vi "OdorSystem-V2.1.vi"() -> ()   [LabVIEW 2019]
doc: "Control odor delivery system in Setup B\n\nNeeds Labview 2019 and DAQmx 19! So that it is compatible with scanimage on Setup B\n\nBy Dr. Jan Eckhardt, Group Friedrich, FMI Basel"
uses:
  StatesEnum.ctl
  <vilib>/Utility/error.llb/DialogType.ctl
  <vilib>/DAQmx/write.llb/DAQmx Write (Digital 1D Bool NChan 1Samp 1Line).vi
  <vilib>/DAQmx/write.llb/DAQmx Write (Digital Wfm 1Chan NSamp).vi
  <vilib>/DAQmx/read.llb/DAQmx Read (Counter U32 1Chan 1Samp).vi
  <vilib>/DAQmx/read.llb/DAQmx Read (Digital 1D Bool 1Chan 1Samp).vi
  <vilib>/Utility/config.llb/Read Key (Double).vi
  <vilib>/Utility/config.llb/Read Key (I32).vi
  <vilib>/Utility/config.llb/Read Key (Boolean).vi
  <vilib>/Utility/config.llb/Read Key (String).vi
  <vilib>/DAQmx/miscellaneous.llb/DAQmx Fill In Error Info.vi
  <vilib>/DAQmx/create/channels.llb/DAQmx Create Channel (CO-Pulse Generation-Frequency).vi
  <vilib>/Waveform/DWDTOps.llb/Digital Pattern Generator (Single Value).vi
  <vilib>/Waveform/DWDTOps.llb/DWDT Append Digital Samples.vi
  <vilib>/DAQmx/configure/timing.llb/DAQmx Timing (Implicit).vi
  <vilib>/DAQmx/create/channels.llb/DAQmx Create Channel (CI-Count Edges).vi
  <vilib>/DAQmx/configure/timing.llb/DAQmx Timing (Sample Clock).vi
  <vilib>/Waveform/DWDTOps.llb/DWDT Append Digital Signals.vi
  <vilib>/Waveform/DWDTOps.llb/DWDT Digital to Boolean Array.vi
  <vilib>/DAQmx/create/channels.llb/DAQmx Create Channel (DO-Digital Output).vi
  <vilib>/Waveform/DWDTOps.llb/DWDT Uncompress Digital.vi
  <resource>/objmgr/daqmx.rc
  <vilib>/Utility/config.llb/NI_LVConfig.lvlib
panel:
  out "Loaded experiment":string
  in  "Load exp. ini":bool
  in  "Use Default valve":bool=TRUE
  in  "Selected default valve":u8(knob)=8 min=1 max=8 step=1 scale=1.0..8.0
  out "Framecount":u32
  in  "Image count filepath":path
  out "Experiment running":bool
  out "State":T1
  in  "Select experiment":enum32{"Single trial", "Trial series"}(tab)
  out "Time elapsed":dbl format="%.1f"
  in  "Start single trial":bool
  out "single trial done":bool
  in  "Select valve":u8(knob)=1 min=1 max=8 step=1 scale=1.0..8.0
  out "Pause elapsed time":dbl format="%#.1f"
  out "In between trials":bool
  out "Trial elapsed time":dbl format="%.1f"
  out "Total elapsed time":dbl format="%.1f"
  out "Estimated total time":dbl
  out "Current list index":i32
  out "Current Valve":u8
  in  "Time between trials":u16=10 min=1 max=900 step=1
  in  "Start trial series":bool
  in  "Valve order list":i8[](array[numeric]) min=1 max=8 step=1
  out "Digitaler output":digitalwaveform(graph)
  out "Stop Boolesch":bool
  in  "Total trial time":dbl=20.0 min=1.0 step=0.1
  in  "Valve opening time":dbl=10.0 min=0.0 step=0.1
  in  "Valve delay":dbl=2.0 min=0.0 step=0.1
  in  "Stopp":bool
  out "Digital Waveform Graph":digitalwaveform(graph)
  # "All times are in second!"
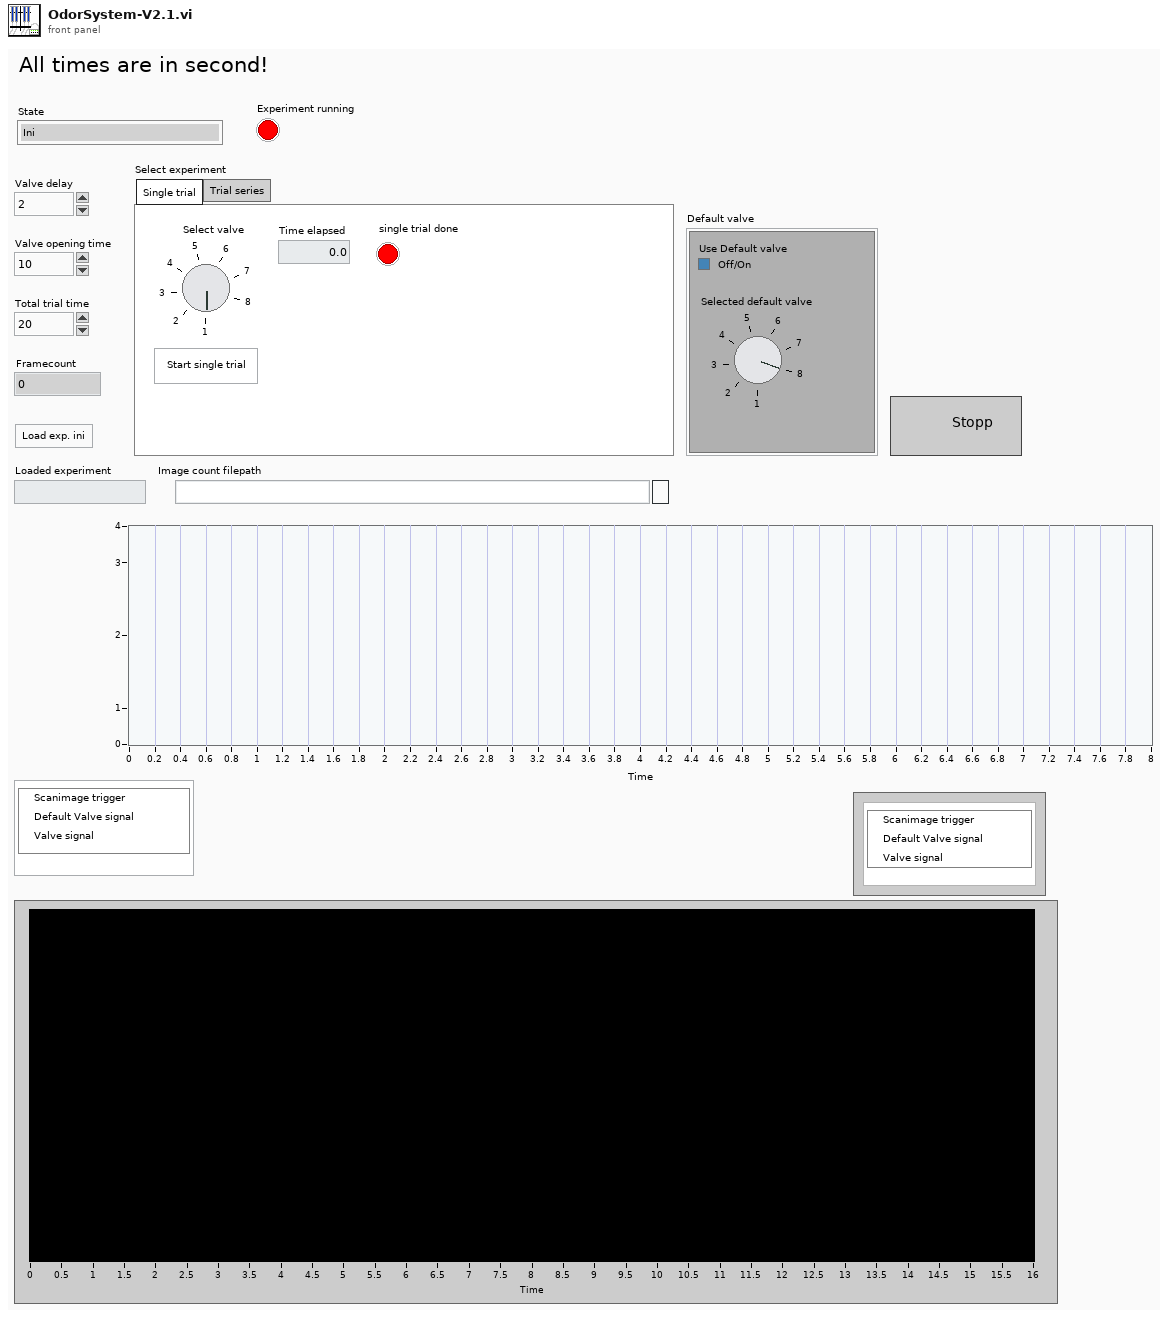
[diagram p1: front panel]
types:
  T1 = typedef "StatesEnum.ctl" = enum16{"Ini", "Standby", "Start Trial", "Start trial series", "Stop"}
  T2 = enum8{"Enabled", "Disabled", "Disabled and Grayed Out"}
  T3 = enum32{"Page Enabled", "Page Disabled", "Page Disabled & Grayed"}
  T4 = typedef "NI_LVConfig.lvlib/Config Data RefNum.ctl" = refnum<k1>
  T5 = typedef "DialogType.ctl" = u16
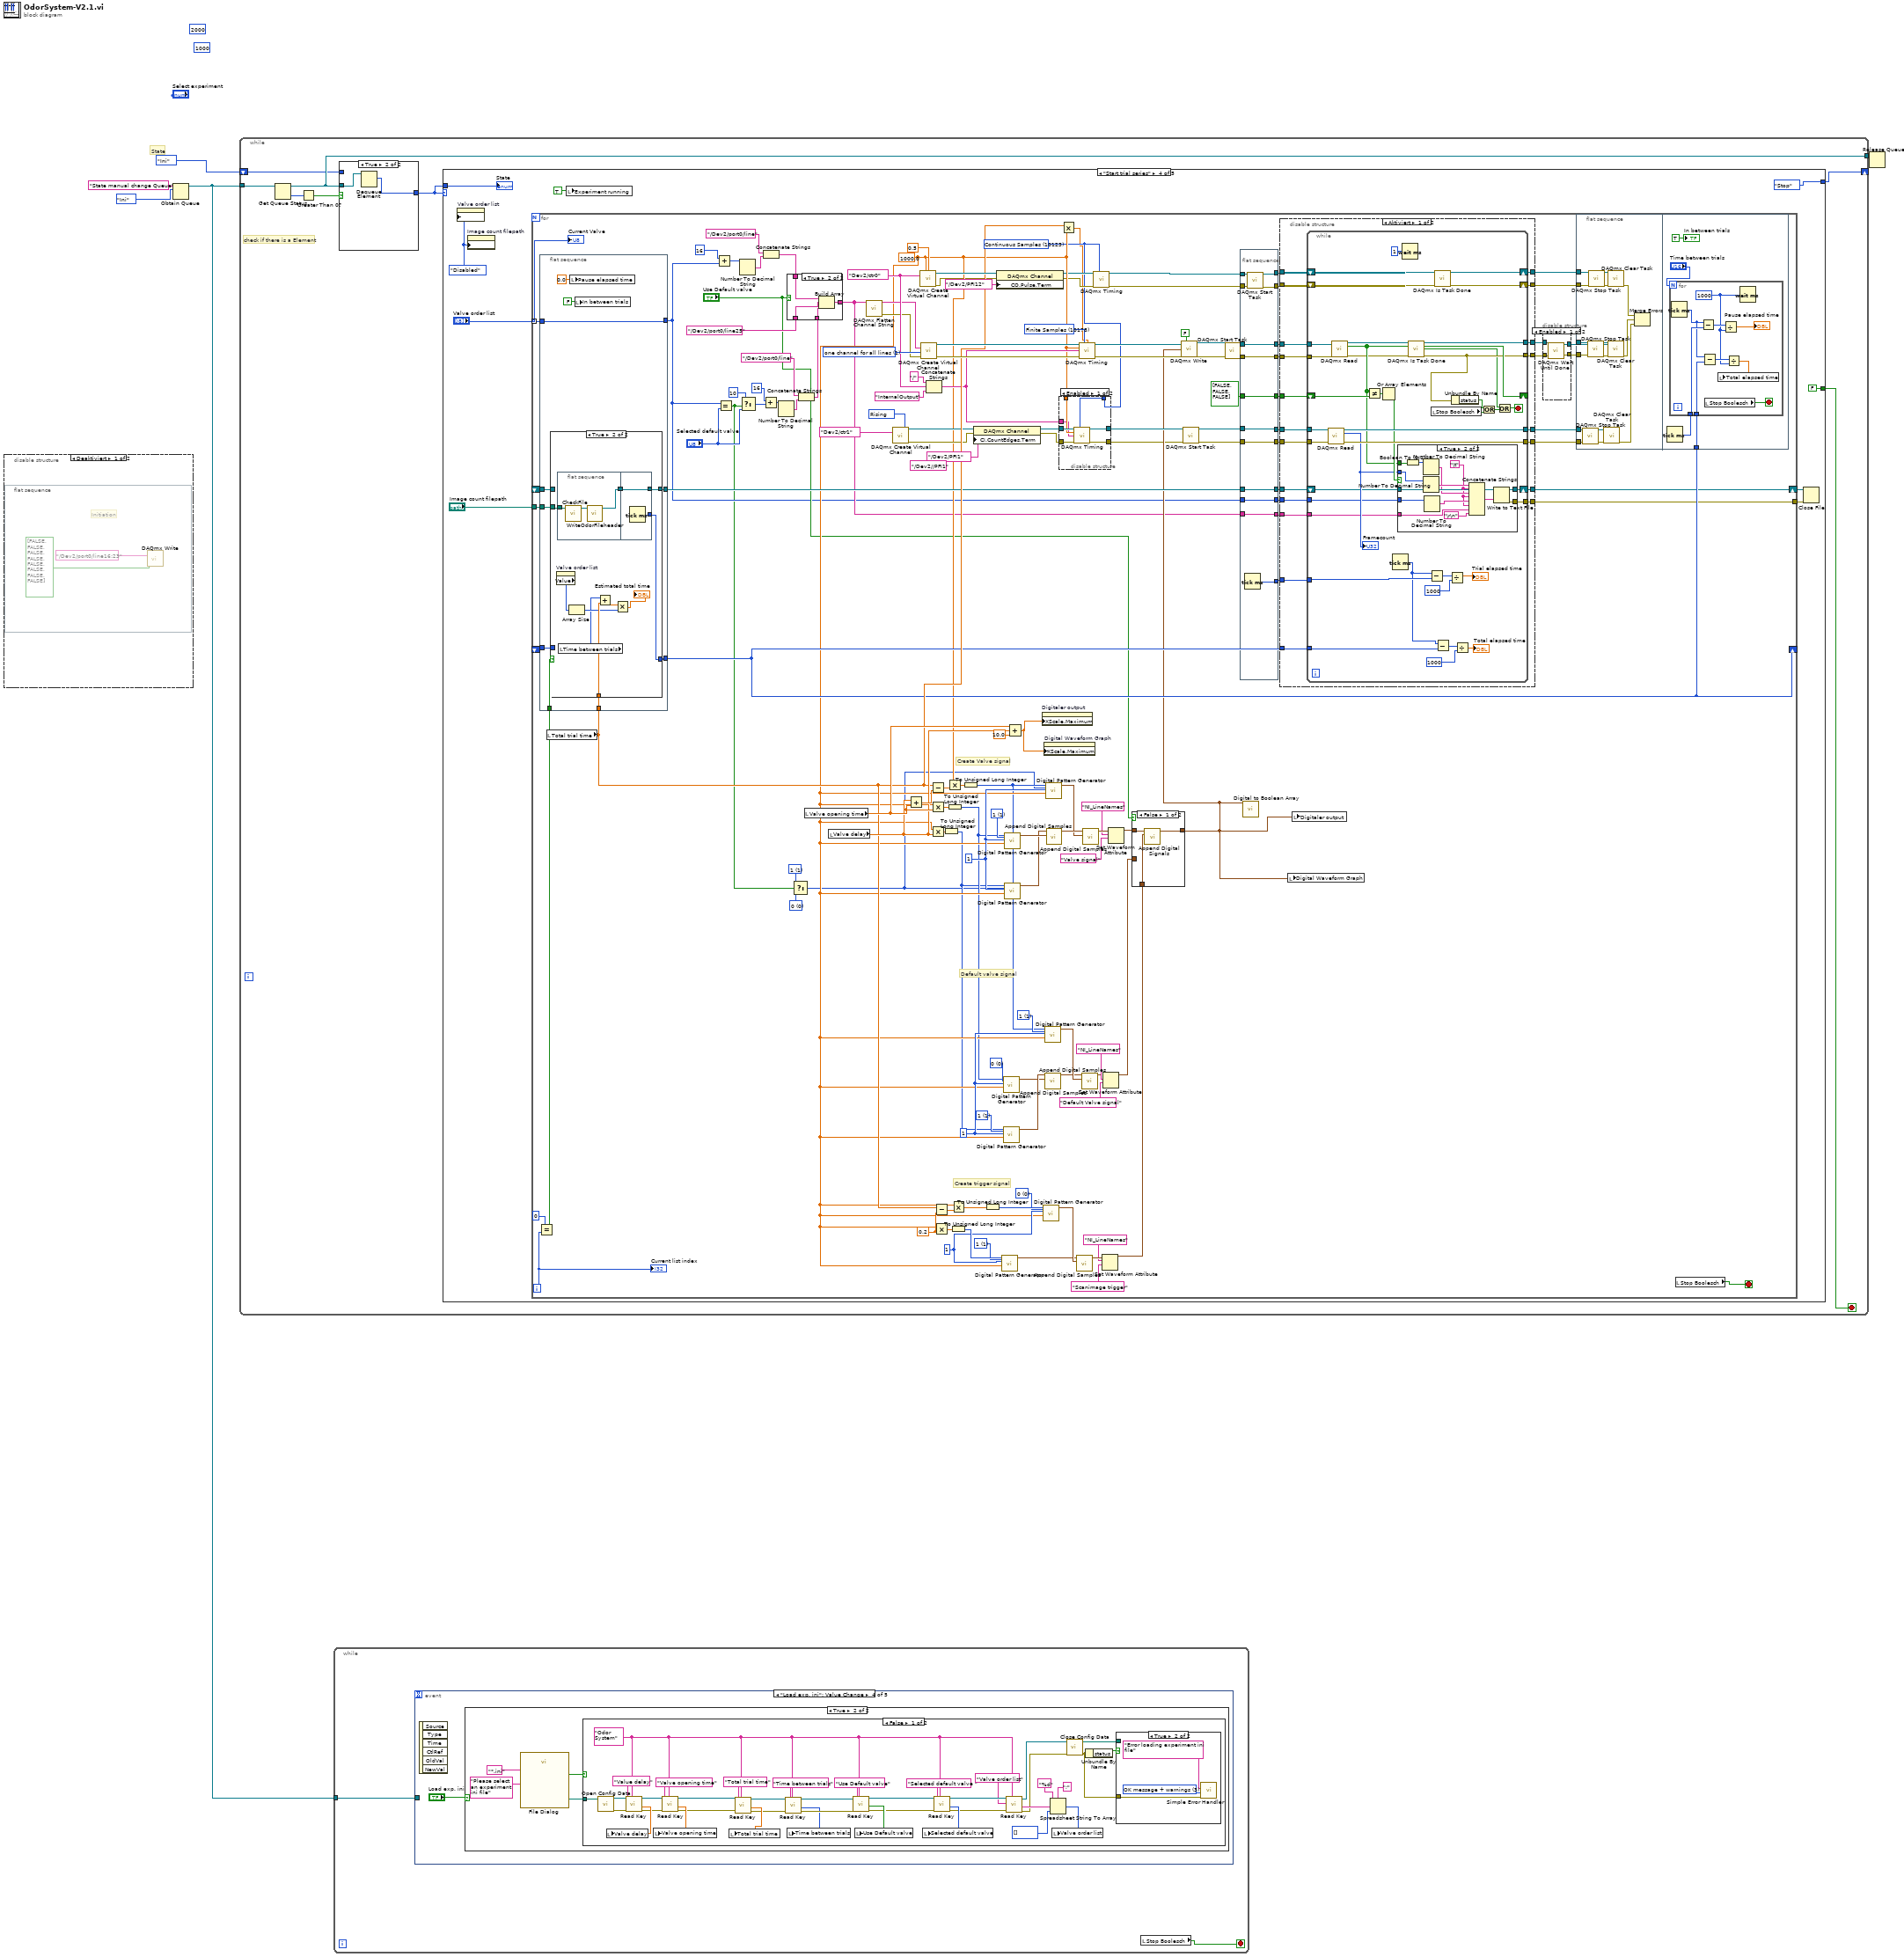
[diagram p0: block diagram]
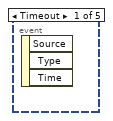
[diagram p3: hidden frame]
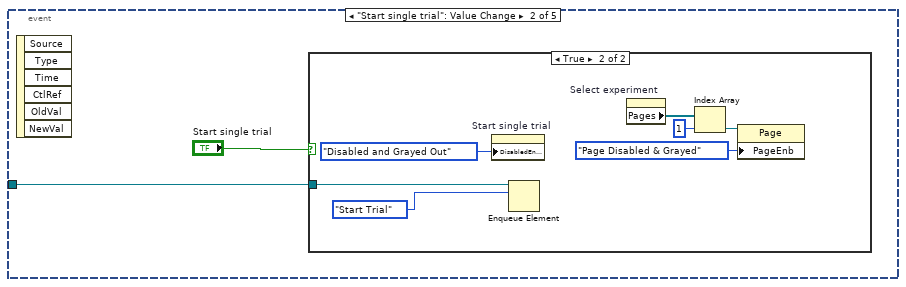
[diagram p4: hidden frame]
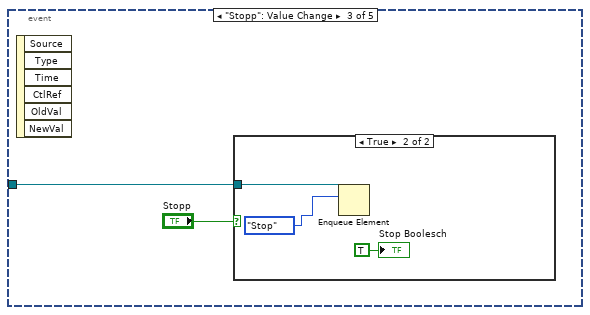
[diagram p6: hidden frame]
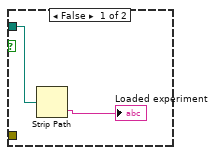
[diagram p9: hidden frame]
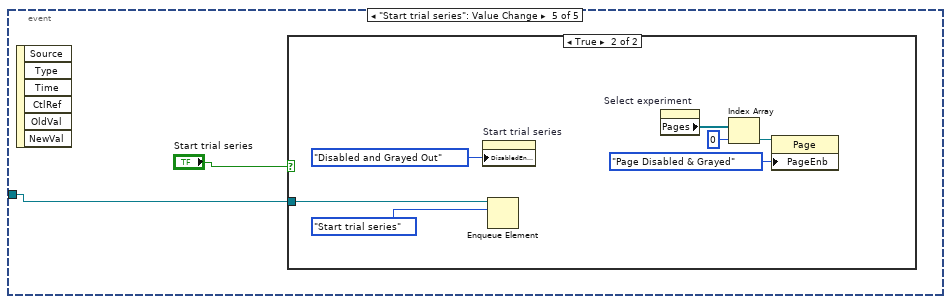
[diagram p11: hidden frame]
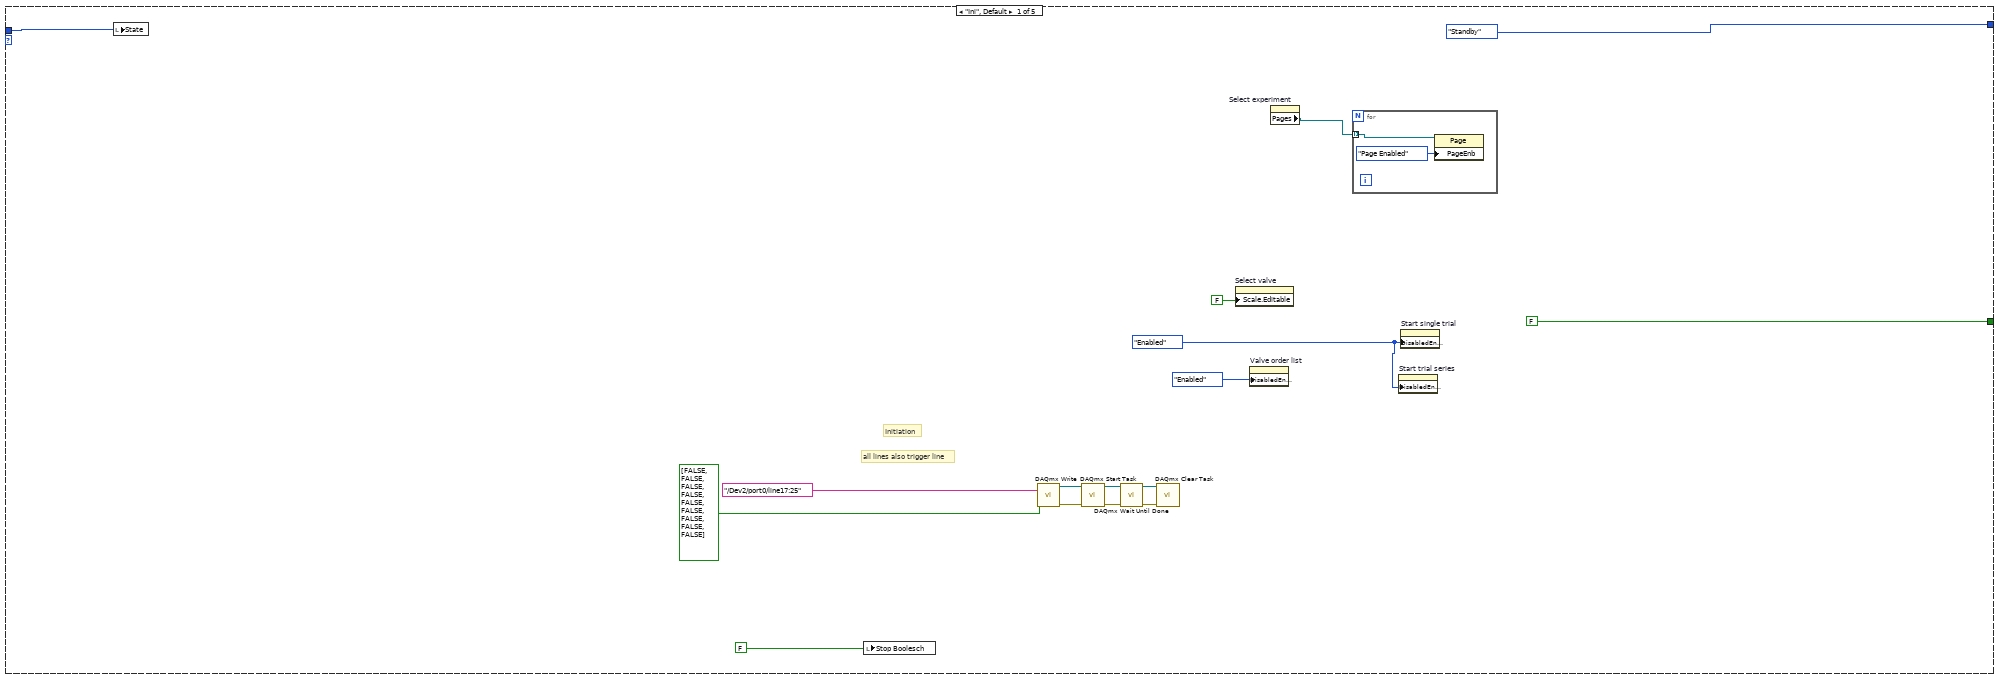
[diagram p14: hidden frame]
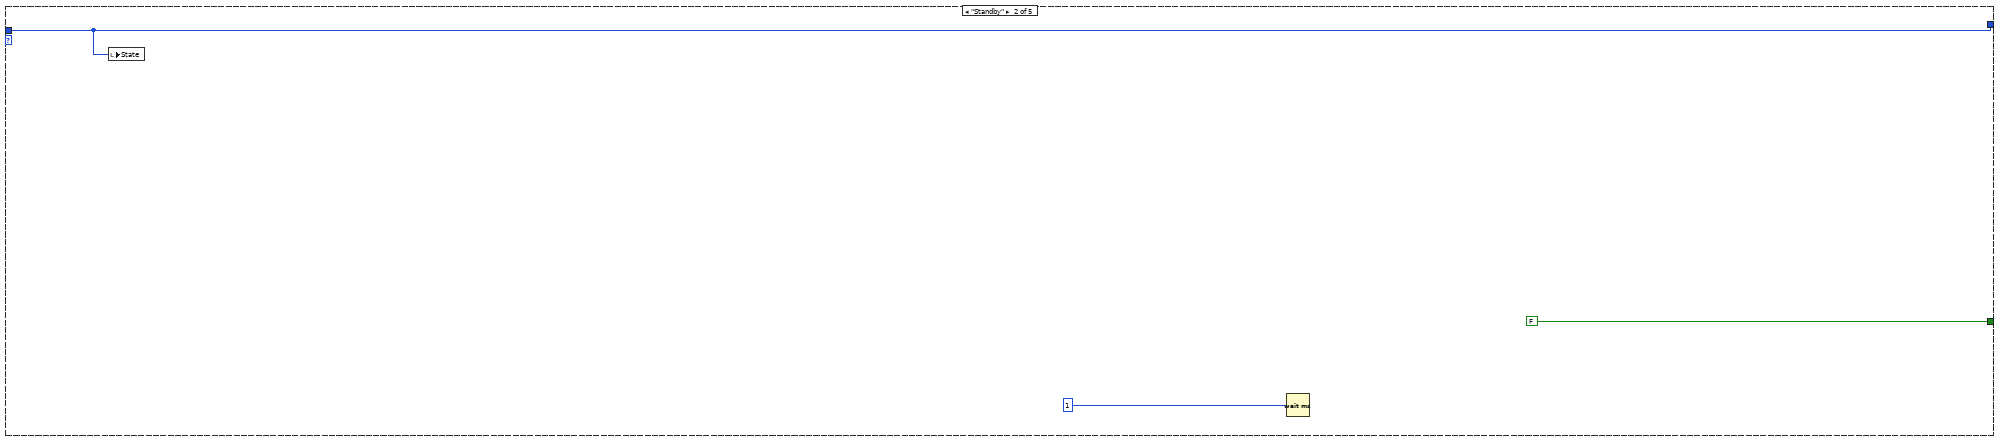
[diagram p15: hidden frame]
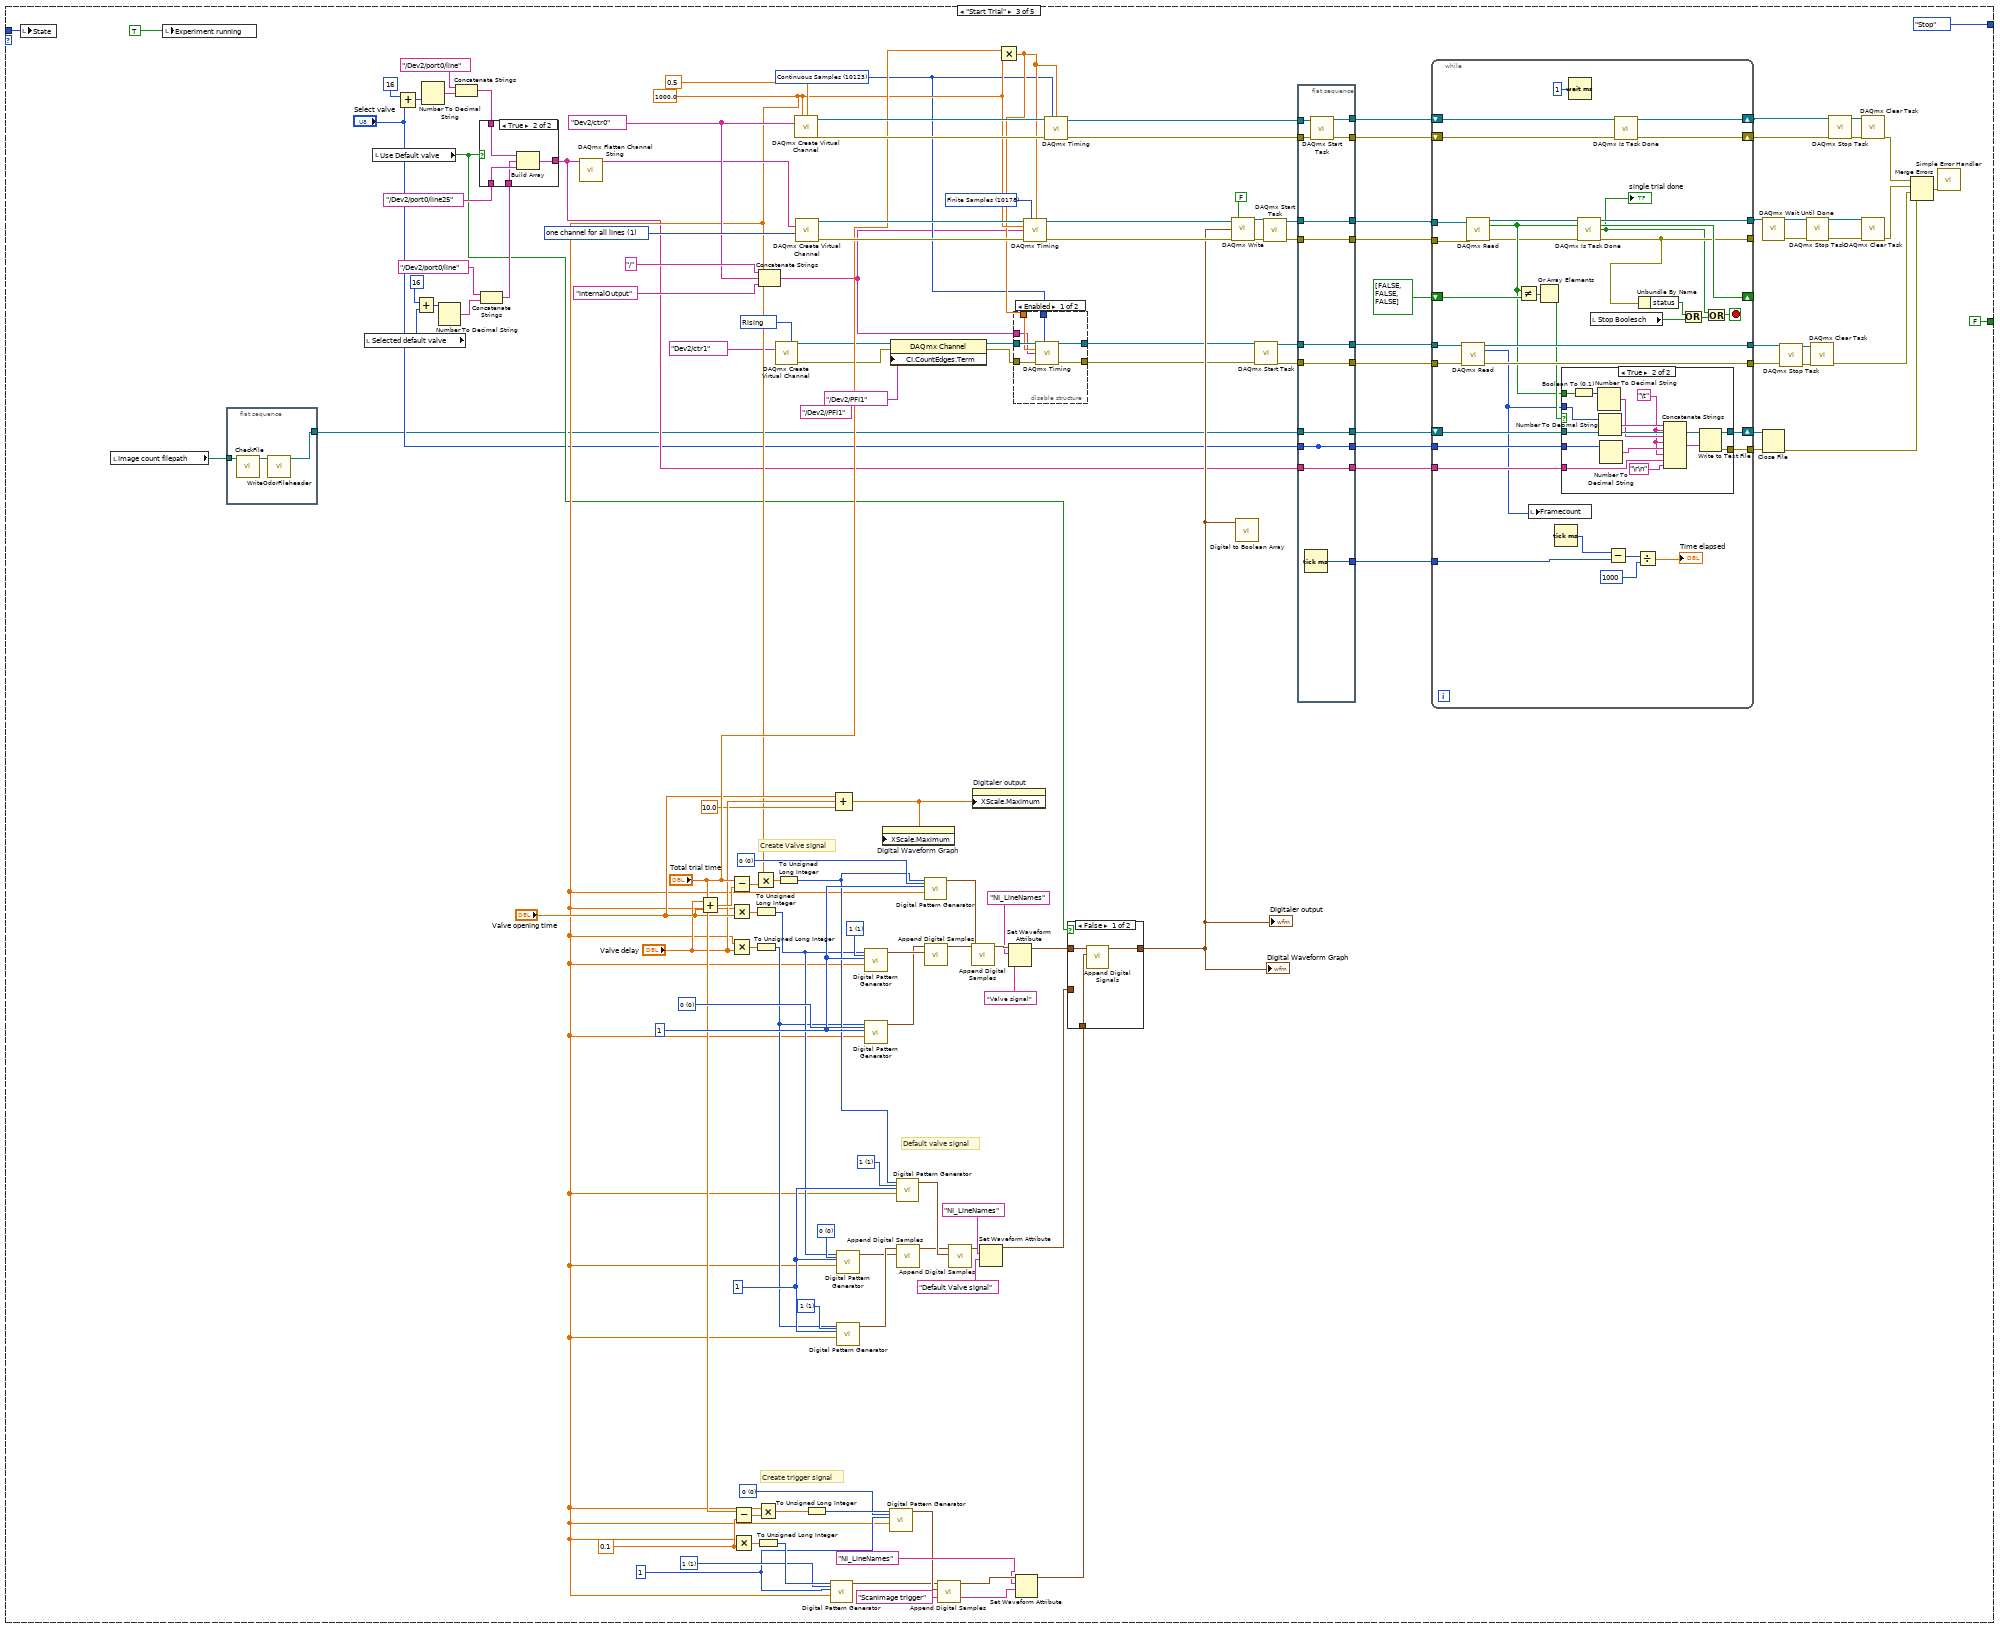
[diagram p16: hidden frame]
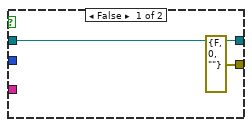
[diagram p17: hidden frame]
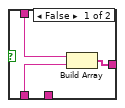
[diagram p18: hidden frame]
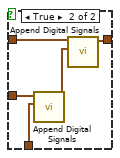
[diagram p20: hidden frame]
diagram:
  (unwired) u32 2000 ("number of samples")
  (unwired) u32 1000 ("number of samples")
  # "State"
  n1 = disable-structure shown="Deaktiviert" {
    frame Disabled {
      n2 = flat-sequence {
        frame #0 {
          # "Initiation"
          n3 = call-poly <vilib>:"DAQmx Write.vi"("task/channels in"="/Dev2/port0/line16:23" ("string"), "data"=bool[] [FALSE, FALSE, FALSE, FALSE, FALSE, FALSE, FALSE, FALSE]) -> ()  [unwired: 11 in, 3 out]
        }
      }
    }
    frame Enabled {
    }
  }
  n4 = Obtain Queue(name (unnamed)="State manual change Queue", element data type=StatesEnum."Ini" ("Enum")) -> (queue out=w4:refnum<queue>)  [unwired: 3 in, 2 out]
  n5 = while {
    tunnel: w4 -> [w13]
    tunnel: [w12] -> w3
    shift-right: [w8] -> _
    shift-left: StatesEnum."Ini" -> [w9]
    stop <- w11 stop-if-true
    # "check if there is a Element"
    n6 = Get Queue Status(queue=w13) -> (queue out=w12:refnum<queue>, # elements in queue=w15:i32)  [unwired: 2 in, 6 out]
    n7 = Greater Than 0?(x=w15) -> (x > 0?=w14:bool)
    n8 = case shown="True" w14 {
      tunnel: w12 -> [_ w18]
      tunnel: w9 -> [w16 _]
      tunnel: [w16 w17] -> w10
      frame False {
      }
      frame True {
        n9 = Dequeue Element(queue=w18) -> (element=w17:T1)  [unwired: 2 in, 3 out]
      }
    }
    n10 = case shown="\"Start trial series\"" w10 {
      tunnel: w10 -> [w29 w37 w115 w276 w595]
      tunnel: [FALSE ("Stop Boolesch") FALSE ("Stop Boolesch") FALSE ("Stop Boolesch") FALSE ("Stop Boolesch") w597] -> w11
      tunnel: [StatesEnum."Standby" ("Enum") w37 StatesEnum."Stop" ("Enum") StatesEnum."Stop" ("Enum") StatesEnum."Standby" ("Enum")] -> w8
      frame "Ini", Default {
        w22 = T2."Enabled" ("Deaktiviert")
        # "all lines also trigger line"
        # "Initiation"
        n11 = local write "State"(w29) -> ()
        n12 = local write "Stop Boolesch"(FALSE ("Stop Boolesch")) -> ()
        n13 = call-poly <vilib>:"DAQmx Write.vi"("task/channels in"="/Dev2/port0/line17:25" ("string"), "data"=bool[] [FALSE, FALSE, FALSE, FALSE, FALSE, FALSE, FALSE, FALSE, FALSE]) -> ("task out"=w24:refnum<k21>, "error out"=w23:errorcluster)  [unwired: 11 in, 1 out]
        n14 = call <vilib>:"DAQmx Start Task.vi"("task/channels in"=w24, "error in"=w23) -> ("task out"=w28:refnum<k21>, "error out"=w26:errorcluster)  [unwired: 12 in]
        n15 = call <vilib>:"DAQmx Wait Until Done.vi"("task/channels in"=w28, "error in"=w26) -> ("task out"=w27:refnum<k21>, "error out"=w25:errorcluster)  [unwired: 12 in]
        n16 = call <vilib>:"DAQmx Clear Task.vi"("task in"=w27, "error in"=w25) -> ()  [unwired: 13 in, 1 out]
        n17 = property on="Select valve" class="Knob (strict)"("Scale.Editable"=FALSE ("Skala.Editierbar")) -> ()  [unwired: 2 in, 2 out]
        n18 = property on="Valve order list" class="Arr (strict)"("DisabledEnum"=T2."Enabled" ("Deaktiviert")) -> ()  [unwired: 2 in, 2 out]
        n19 = property on="Select experiment" class="TabCtl (strict)"() -> ("Pages"=w20:refnum<vi>[])  [unwired: 2 in, 2 out]
        n20 = for {
          tunnel: w20 -> [w35] mode=indexing
          n21 = property class="Page"(reference=w35, "PageEnb"=T3."Page Enabled" ("Aktiv-Status der Seite")) -> ()  [unwired: 1 in, 2 out]
        }
        n22 = property on="Start trial series" class="Bool"("DisabledEnum"=w22) -> ()  [unwired: 2 in, 2 out]
        n23 = property on="Start single trial" class="Bool"("DisabledEnum"=w22) -> ()  [unwired: 2 in, 2 out]
      }
      frame "Standby" {
        n24 = local write "State"(w37) -> ()
        n25 = Wait (ms)(milliseconds to wait=u32 1 ("Zu wartende ms")) -> ()  [unwired: 1 out]
      }
      frame "Start Trial" {
        w83 = 10178 items=["Finite Samples"=10178, "Continuous Samples"=10123, "Hardware Timed Single Point"=12522] ("sample mode")
        (unwired) "/Dev2//PFI1" ("string")
        w93 = 10280 items=["Rising"=10280, "Falling"=10171] ("edge")
        w103 = u32 1 ("number of signals")
        w106 = u8 1 items=["0", "1", "Z", "L", "H", "X", "T", "V"] ("value")
        w105 = u8 0 items=["0", "1", "Z", "L", "H", "X", "T", "V"] ("value")
        w104 = u8 1 items=["0", "1", "Z", "L", "H", "X", "T", "V"] ("value")
        w135 = 0.1 ("y")
        w138 = u32 1 ("number of signals")
        w140 = u8 0 items=["0", "1", "Z", "L", "H", "X", "T", "V"] ("value")
        w139 = u8 1 items=["0", "1", "Z", "L", "H", "X", "T", "V"] ("value")
        w155 = tag "Dev2/ctr0" ("counter")
        w99 = 1000.0 ("frequency")
        w159 = u32 1 ("number of signals")
        w160 = u8 0 items=["0", "1", "Z", "L", "H", "X", "T", "V"] ("value")
        w161 = u8 1 items=["0", "1", "Z", "L", "H", "X", "T", "V"] ("value")
        w162 = u8 0 items=["0", "1", "Z", "L", "H", "X", "T", "V"] ("value")
        w173 = 1 items=["one channel for each line", "one channel for all lines"] ("line grouping")
        w84 = 10123 items=["Finite Samples"=10178, "Continuous Samples"=10123] ("sample mode")
        # "Default valve signal"
        # "Create trigger signal"
        # "Create Valve signal"
        n26 = local write "State"(w115) -> ()
        n27 = local read "Image count filepath"() -> (w54:path)
        n28 = local write "Experiment running"(TRUE ("Experiment running")) -> ()
        n29 = flat-sequence {
          tunnel: w54 -> [w182]
          tunnel: [w180] -> w55
          frame #0 {
            n30 = call "CheckFile.vi"("Image count filepath"=w182) -> ("Byte Stream File out"=w181:refnum<file>)  [unwired: 10 in]
            n31 = call "WriteOdorFileheader.vi"("Byte Stream File in"=w181) -> ("Byte Stream File out"=w180:refnum<file>)  [unwired: 10 in]
          }
        }
        n32 = local read "Selected default valve"() -> (w73:u8)
        n33 = local read "Use Default valve"() -> (w74:bool)
        n34 = Add(x=i8 16, y="Select valve") -> (x+y=w147:u8)
        n35 = Add(x=i8 16, y=w73) -> (x+y=w80:u8)
        n36 = Number To Decimal String(number=w147) -> (decimal integer string=w148:string)  [unwired: 1 in]
        n37 = Number To Decimal String(number=w80) -> (decimal integer string=w79:string)  [unwired: 1 in]
        n38 = Concatenate Strings("/Dev2/port0/line" ("string"), w148) -> (w77:string)
        n39 = Concatenate Strings("/Dev2/port0/line" ("string"), w79) -> (w75:string)
        n40 = case shown="True" w74 {
          tunnel: w77 -> [w236 w239]
          tunnel: "/Dev2/port0/line25" ("string") -> [w235 w238]
          tunnel: [w234 w240] -> w58
          tunnel: w75 -> [_ w237]
          frame False {
            n41 = Build Array(w236, w235) -> (w234:string[])
          }
          frame True {
            n42 = Build Array(w239, w237, w238) -> (w240:string[])
          }
        }
        n43 = call <vilib>:"DAQmx Flatten Channel String.vi"("names in"=w58) -> ("names out"=w137:string)  [unwired: 13 in, 1 out]
        n44 = Add(x="Valve delay", y="Valve opening time") -> (x+y=w151:dbl)
        n45 = Subtract(x="Total trial time", y=w151) -> (x-y=w150:dbl)
        n46 = Multiply(x=w99, y="Valve opening time") -> (x*y=w153:dbl)
        n47 = Multiply(x=w99, y="Valve delay") -> (x*y=w154:dbl)
        n48 = Subtract(x="Total trial time", y=w135) -> (x-y=w145:dbl)
        n49 = Multiply(x=w99, y=w135) -> (x*y=w141:dbl)
        n50 = Multiply(x=w99, y=w150) -> (x*y=w152:dbl)
        n51 = To Unsigned Long Integer(number=w153) -> (unsigned 32bit integer=w101:u32)
        n52 = To Unsigned Long Integer(number=w154) -> (unsigned 32bit integer=w100:u32)
        n53 = Multiply(x=w99, y=w145) -> (x*y=w143:dbl)
        n54 = To Unsigned Long Integer(number=w141) -> (unsigned 32bit integer=w142:u32)
        n55 = Concatenate Strings("/", w155, "InternalOutput" ("string")) -> (w82:string)
        n56 = call-poly <vilib>:"DAQmx Create Virtual Channel.vi"("edge"=w93, "counter"=tag "Dev2/ctr1") -> ("task out"=w91:refnum<k21>, "error out"=w88:errorcluster)  [unwired: 12 in]
        n57 = To Unsigned Long Integer(number=w152) -> (unsigned 32bit integer=w102:u32)
        n58 = call-poly <vilib>:"DAQmx Create Virtual Channel.vi"("frequency"=w99, "duty cycle"=0.5, "counter"=w155) -> ("task out"=w176:refnum<k21>, "error out"=w177:errorcluster)  [unwired: 11 in]
        n59 = call-poly <vilib>:"DAQmx Create Virtual Channel.vi"("lines"=w137, "line grouping"=w173) -> ("task out"=w179:refnum<k21>, "error out"=w178:errorcluster)  [unwired: 12 in]
        n60 = To Unsigned Long Integer(number=w143) -> (unsigned 32bit integer=w144:u32)
        n61 = call-poly <vilib>:"Digital Pattern Generator.vi"("value"=w139, "sample rate"=w99, "number of signals"=w138, "number of samples"=w142) -> ("digital waveform"=w123:digitalwaveform)  [unwired: 6 in, 1 out]
        n62 = Compound Arithmetic op=ADD("Valve opening time", "Valve delay", 10.0 ("Wert")) -> (w116:dbl)
        n63 = call-poly <vilib>:"Digital Pattern Generator.vi"("value"=w105, "sample rate"=w99, "number of signals"=w103, "number of samples"=w101) -> ("digital waveform"=w110:digitalwaveform)  [unwired: 6 in, 1 out]
        n64 = call-poly <vilib>:"Digital Pattern Generator.vi"("value"=w104, "sample rate"=w99, "number of signals"=w103, "number of samples"=w100) -> ("digital waveform"=w111:digitalwaveform)  [unwired: 6 in, 1 out]
        n65 = call-poly <vilib>:"Digital Pattern Generator.vi"("value"=w161, "sample rate"=w99, "number of signals"=w159, "number of samples"=w101) -> ("digital waveform"=w128:digitalwaveform)  [unwired: 6 in, 1 out]
        n66 = call-poly <vilib>:"Digital Pattern Generator.vi"("value"=w162, "sample rate"=w99, "number of signals"=w159, "number of samples"=w100) -> ("digital waveform"=w127:digitalwaveform)  [unwired: 6 in, 1 out]
        n67 = property on="Digital Waveform Graph" class="DigitalGraph (strict)"("XScale.Maximum"=w116) -> ()  [unwired: 2 in, 2 out]
        n68 = call-poly <vilib>:"Digital Pattern Generator.vi"("value"=w140, "sample rate"=w99, "number of signals"=w138, "number of samples"=w144) -> ("digital waveform"=w124:digitalwaveform)  [unwired: 6 in, 1 out]
        n69 = property class="DAQmx Channel"(reference=w91, error in=w88, "CI.CountEdges.Term"=tag "/Dev2/PFI1") -> (reference out=w90:refnum<k21>, error out=w89:errorcluster)
        n70 = call-poly <vilib>:"Digital Pattern Generator.vi"("value"=w106, "sample rate"=w99, "number of signals"=w103, "number of samples"=w102) -> ("digital waveform"=w113:digitalwaveform)  [unwired: 6 in, 1 out]
        n71 = call-poly <vilib>:"Append Digital Samples.vi"("digital waveform B"=w110, "digital waveform A"=w111) -> ("digital waveform out"=w112:digitalwaveform)  [unwired: 8 in, 1 out]
        n72 = call-poly <vilib>:"Digital Pattern Generator.vi"("value"=w160, "sample rate"=w99, "number of signals"=w159, "number of samples"=w102) -> ("digital waveform"=w125:digitalwaveform)  [unwired: 6 in, 1 out]
        n73 = call-poly <vilib>:"Append Digital Samples.vi"("digital waveform B"=w128, "digital waveform A"=w127) -> ("digital waveform out"=w126:digitalwaveform)  [unwired: 8 in, 1 out]
        n74 = call-poly <vilib>:"Append Digital Samples.vi"("digital waveform B"=w124, "digital waveform A"=w123) -> ("digital waveform out"=w134:digitalwaveform)  [unwired: 8 in, 1 out]
        n75 = call-poly <vilib>:"Append Digital Samples.vi"("digital waveform B"=w113, "digital waveform A"=w112) -> ("digital waveform out"=w107:digitalwaveform)  [unwired: 8 in, 1 out]
        n76 = call-poly <vilib>:"Append Digital Samples.vi"("digital waveform B"=w125, "digital waveform A"=w126) -> ("digital waveform out"=w131:digitalwaveform)  [unwired: 8 in, 1 out]
        n77 = property on="Digitaler output" class="DigitalGraph (strict)"("XScale.Maximum"=w116) -> ()  [unwired: 2 in, 2 out]
        n78 = Set Waveform Attribute(5:"Default Valve signal", 6:"NI_LineNames" ("name"), 7:w107) -> (3:w95:digitalwaveform)  [unwired: 1 in, 2 out]
        n79 = Multiply(x="Total trial time", y=w99) -> (x*y=w85:dbl)
        n80 = Set Waveform Attribute(5:"Valve signal", 6:"NI_LineNames" ("name"), 7:w131) -> (3:w98:digitalwaveform)  [unwired: 1 in, 2 out]
        n81 = disable-structure shown="Enabled" {
          disable-tunnel: w90 -> [w247 w249]
          disable-tunnel: w85 -> [w246 _]
          disable-tunnel: w82 -> [w245 _]
          disable-tunnel: w89 -> [w244 w248]
          disable-tunnel: [w243 w249] -> w92
          disable-tunnel: [w242 w248] -> w86
          disable-tunnel: w84 -> [w241 _]
          frame Enabled {
            n82 = call-poly <vilib>:"DAQmx Timing.vi"("task/channels in"=w247, "sample mode"=w241, "rate"=w246, "source"=w245, "error in"=w244) -> ("task out"=w243:refnum<k21>, "error out"=w242:errorcluster)  [unwired: 9 in]
          }
          frame Disabled {
          }
        }
        n83 = Set Waveform Attribute(5:"Scanimage trigger", 6:"NI_LineNames" ("name"), 7:w134) -> (3:w96:digitalwaveform)  [unwired: 1 in, 2 out]
        n84 = call-poly <vilib>:"DAQmx Timing.vi"("task/channels in"=w179, "sample mode"=w83, "samples per channel"=w85, "rate"=w99, "source"=w82, "error in"=w178) -> ("task out"=w170:refnum<k21>, "error out"=w169:errorcluster)  [unwired: 8 in]
        n85 = call-poly <vilib>:"DAQmx Timing.vi"("task/channels in"=w176, "sample mode"=w84, "samples per channel"=w85, "error in"=w177) -> ("task out"=w174:refnum<k21>, "error out"=w175:errorcluster)  [unwired: 10 in]
        n86 = case shown="False" w74 {
          tunnel: w98 -> [w252 w257]
          tunnel: w96 -> [w251 w255]
          tunnel: [w250 w256] -> w97
          tunnel: w95 -> [_ w254]
          frame False {
            n87 = call-poly <vilib>:"Append Digital Signals.vi"("digital waveform (low bits)"=w251, "digital waveform (high bits)"=w252) -> ("digital waveform out"=w250:digitalwaveform)  [unwired: 8 in, 1 out]
          }
          frame True {
            n88 = call-poly <vilib>:"Append Digital Signals.vi"("digital waveform (low bits)"=w255, "digital waveform (high bits)"=w254) -> ("digital waveform out"=w253:digitalwaveform)  [unwired: 8 in, 1 out]
            n89 = call-poly <vilib>:"Append Digital Signals.vi"("digital waveform (low bits)"=w253, "digital waveform (high bits)"=w257) -> ("digital waveform out"=w256:digitalwaveform)  [unwired: 8 in, 1 out]
          }
        }
        "Digital Waveform Graph" <- w97
        "Digitaler output" <- w97
        n90 = call-poly <vilib>:"DAQmx Write.vi"("task/channels in"=w170, "auto start"=FALSE, "data"=w97, "error in"=w169) -> ("task out"=w168:refnum<k21>, "error out"=w167:errorcluster)  [unwired: 9 in, 1 out]
        n91 = call-poly <vilib>:"Digital to Boolean Array.vi"("digital waveform"=w97) -> ()  [unwired: 9 in, 2 out]
        n92 = call <vilib>:"DAQmx Start Task.vi"("task/channels in"=w92, "error in"=w86) -> ("task out"=w66:refnum<k21>, "error out"=w65:errorcluster)  [unwired: 12 in]
        n93 = call <vilib>:"DAQmx Start Task.vi"("task/channels in"=w168, "error in"=w167) -> ("task out"=w172:refnum<k21>, "error out"=w171:errorcluster)  [unwired: 12 in]
        n94 = flat-sequence {
          tunnel: [w269] -> w72
          tunnel: [w268] -> w71
          tunnel: w175 -> [w267]
          tunnel: w174 -> [w266]
          tunnel: [w265] -> w70
          tunnel: w172 -> [w265]
          tunnel: [w264] -> w69
          tunnel: w171 -> [w264]
          tunnel: [w263] -> w62
          tunnel: [w262] -> w64
          tunnel: w66 -> [w262]
          tunnel: [w261] -> w63
          tunnel: w65 -> [w261]
          tunnel: [w260] -> w61
          tunnel: w58 -> [w260]
          tunnel: [w258] -> w60
          tunnel: [w258] -> _
          tunnel: [w259] -> w59
          tunnel: w55 -> [w259]
          tunnel: "Select valve" -> [w258]
          frame #0 {
            n95 = Tick Count (ms)() -> (millisecond timer value=w263:u32)
            n96 = call <vilib>:"DAQmx Start Task.vi"("task/channels in"=w266, "error in"=w267) -> ("task out"=w269:refnum<k21>, "error out"=w268:errorcluster)  [unwired: 12 in]
          }
        }
        n97 = while {
          shift-right: [w214] -> w68
          shift-left: w72 -> [w216]
          shift-right: [w213] -> w42
          shift-left: w71 -> [w215]
          tunnel: w70 -> [w212]
          tunnel: w69 -> [w203]
          tunnel: [w189] -> w67
          tunnel: [w187] -> _
          tunnel: w62 -> [w208]
          tunnel: w64 -> [w202]
          tunnel: w63 -> [w200]
          tunnel: [w201] -> w50
          tunnel: [w199] -> w49
          shift-right: [w195] -> _
          shift-left: bool[] [FALSE, FALSE, FALSE] ("data") -> [w198]
          shift-right: [w193] -> w53
          shift-left: w59 -> [w194]
          tunnel: w61 -> [w192]
          tunnel: w60 -> [w191]
          tunnel: [w190] -> w52
          stop <- w209 stop-if-true
          n98 = call-poly <vilib>:"DAQmx Read.vi"("task/channels in"=w202, "error in"=w200) -> ("task out"=w201:refnum<k21>, "data"=w183:u32, "error out"=w199:errorcluster)  [unwired: 11 in]
          n99 = call-poly <vilib>:"DAQmx Read.vi"("task/channels in"=w212, "error in"=w203) -> ("task out"=w204:refnum<k21>, "data"=w195:bool[], "error out"=w188:errorcluster)  [unwired: 11 in]
          n100 = Not Equal?(x=w195, y=w198) -> (x != y?=w197:bool[])
          n101 = local write "Framecount"(w183) -> ()
          n102 = Or Array Elements(Boolean array=w197) -> (logical OR=w196:bool)
          n103 = Tick Count (ms)() -> (millisecond timer value=w207:u32)
          n104 = case shown="True" w196 {
            tunnel: w195 -> [_ w230]
            tunnel: w183 -> [_ w228]
            tunnel: w194 -> [w219 w232]
            tunnel: [w219 w231] -> w193
            tunnel: w192 -> [_ w222]
            tunnel: w191 -> [_ w225]
            tunnel: [errorcluster {"status"=FALSE, "code"=0, "source"=""} ("error out") w221] -> w190
            frame False {
            }
            frame True {
              w223 = "\t"
              n105 = Boolean To (0,1)(Boolean=w230) -> (0, 1=w229:i16[])
              n106 = Number To Decimal String(number=w229) -> (decimal integer string=w226:string[])  [unwired: 1 in]
              n107 = Number To Decimal String(number=w228) -> (decimal integer string=w227:string)  [unwired: 1 in]
              n108 = Number To Decimal String(number=w225) -> (decimal integer string=w224:string)  [unwired: 1 in]
              n109 = Concatenate Strings(w227, w223, w226, w223, w224, w223, w222, "\r\n") -> (w233:string)
              n110 = Write to Text File(file (use dialog)=w232, text=w233) -> (refnum out=w231:refnum<file>, error out=w221:errorcluster)  [unwired: 2 in, 1 out]
            }
          }
          n111 = Wait (ms)(milliseconds to wait=u32 1 ("Zu wartende ms")) -> ()  [unwired: 1 out]
          n112 = call <vilib>:"DAQmx Is Task Done.vi"("task/channels in"=w204, "error in"=w188) -> ("task out"=w189:refnum<k21>, "task done?"=w185:bool, "error out"=w187:errorcluster)  [unwired: 11 in]
          "single trial done" <- w185
          n113 = local read "Stop Boolesch"() -> (w186:bool)
          n114 = Subtract(x=w207, y=w208) -> (x-y=w206:u32)
          n115 = call <vilib>:"DAQmx Is Task Done.vi"("task/channels in"=w216, "error in"=w215) -> ("task out"=w214:refnum<k21>, "error out"=w213:errorcluster)  [unwired: 11 in, 1 out]
          n116 = Divide(x=w206, y=u32 1000 ("x")) -> (x/y=→"Time elapsed":dbl)
          n117 = Unbundle By Name(w187) -> ("status"=w210:bool)
          n118 = Or(x=w210, y=w186) -> (x .or. y?=w217:bool)
          n119 = Or(x=w185, y=w217) -> (x .or. y?=w209:bool)
        }
        n120 = call <vilib>:"DAQmx Wait Until Done.vi"("task/channels in"=w67) -> ("task out"=w119:refnum<k21>, "error out"=w45:errorcluster)  [unwired: 13 in]
        n121 = Close File(refnum=w53, error in=w52) -> (error out=w40:errorcluster)  [unwired: 1 out]
        n122 = call <vilib>:"DAQmx Stop Task.vi"("task/channels in"=w50, "error in"=w49) -> ("task out"=w51:refnum<k21>, "error out"=w48:errorcluster)  [unwired: 12 in]
        n123 = call <vilib>:"DAQmx Stop Task.vi"("task/channels in"=w119, "error in"=w45) -> ("task out"=w46:refnum<k21>, "error out"=w44:errorcluster)  [unwired: 12 in]
        n124 = call <vilib>:"DAQmx Clear Task.vi"("task in"=w51, "error in"=w48) -> ("error out"=w47:errorcluster)  [unwired: 13 in]
        n125 = call <vilib>:"DAQmx Stop Task.vi"("task/channels in"=w68, "error in"=w42) -> ("task out"=w43:refnum<k21>, "error out"=w41:errorcluster)  [unwired: 12 in]
        n126 = call <vilib>:"DAQmx Clear Task.vi"("task in"=w43, "error in"=w41) -> ("error out"=w165:errorcluster)  [unwired: 13 in]
        n127 = call <vilib>:"DAQmx Clear Task.vi"("task in"=w46, "error in"=w44) -> ("error out"=w164:errorcluster)  [unwired: 13 in]
        n128 = Merge Errors(w165, w164, w47, w40) -> (w163:errorcluster)
        n129 = call <vilib>:"Simple Error Handler.vi"("error in (no error)"=w163) -> ()  [unwired: 4 in, 5 out]
      }
      frame "Start trial series" {
        w272 = T2."Disabled" ("Deaktiviert")
        n130 = property on="Valve order list" class="Arr (strict)"("DisabledEnum"=w272) -> ()  [unwired: 2 in, 2 out]
        n131 = property on="Image count filepath" class="Path"("DisabledEnum"=w272) -> ()  [unwired: 2 in, 2 out]
        n132 = for {
          tunnel: "Valve order list" -> [w353] mode=indexing
          shift-right: [w349] -> _
          shift-left: _ -> [w351]
          tunnel: "Image count filepath" -> [w334]
          shift-right: [w333] -> w271
          shift-left: _ -> [w332]
          tunnel: [w331] -> w270
          i -> [w358]
          stop <- w362 stop-if-true
          w289 = 10178 items=["Finite Samples"=10178, "Continuous Samples"=10123, "Hardware Timed Single Point"=12522] ("sample mode")
          w316 = u32 1 ("number of signals")
          w319 = u8 1 items=["0", "1", "Z", "L", "H", "X", "T", "V"] ("value")
          w318 = u8 0 items=["0", "1", "Z", "L", "H", "X", "T", "V"] ("value")
          w317 = u8 1 items=["0", "1", "Z", "L", "H", "X", "T", "V"] ("value")
          (unwired) "/Dev2//PFI1" ("string")
          w346 = 10280 items=["Rising"=10280, "Falling"=10171] ("edge")
          w379 = 0.2 ("y")
          w381 = u32 1 ("number of signals")
          w383 = u8 0 items=["0", "1", "Z", "L", "H", "X", "T", "V"] ("value")
          w382 = u8 1 items=["0", "1", "Z", "L", "H", "X", "T", "V"] ("value")
          w398 = tag "Dev2/ctr0" ("counter")
          w315 = 1000.0 ("frequency")
          w405 = u32 1 ("number of signals")
          w282 = u8 1 items=["0", "1", "Z", "L", "H", "X", "T", "V"] ("value")
          w406 = u8 1 items=["0", "1", "Z", "L", "H", "X", "T", "V"] ("value")
          w281 = u8 0 items=["0", "1", "Z", "L", "H", "X", "T", "V"] ("value")
          w414 = 1 items=["one channel for each line", "one channel for all lines"] ("line grouping")
          w293 = 10123 items=["Finite Samples"=10178, "Continuous Samples"=10123] ("sample mode")
          # "Default valve signal"
          # "Create trigger signal"
          # "Create Valve signal"
          n133 = Equal?(x=0, y=w358) -> (x = y?=w352:bool)
          n134 = flat-sequence {
            tunnel: [w461] -> w286
            tunnel: w353 -> [w461]
            tunnel: w352 -> [w460]
            tunnel: w351 -> [w459]
            tunnel: w350 -> [w458]
            tunnel: [w457] -> w349
            tunnel: [w454] -> w339
            tunnel: w334 -> [w453]
            tunnel: w332 -> [w452]
            frame #0 {
              n135 = case shown="True" w460 {
                tunnel: [w463 w464] -> w457
                tunnel: w459 -> [w463 _]
                tunnel: w458 -> [_ w473]
                tunnel: w453 -> [_ w467]
                tunnel: [w462 w466] -> w454
                tunnel: w452 -> [w462 _]
                frame False {
                }
                frame True {
                  n136 = property on="Valve order list" class="Arr (strict)"() -> ("Value"=w471:i8[])  [unwired: 2 in, 2 out]
                  n137 = flat-sequence {
                    tunnel: w467 -> [w476]
                    tunnel: [w474] -> w465
                    tunnel: [w478] -> w466
                    tunnel: w465 -> [w478]
                    tunnel: [w477] -> w464
                    frame #0 {
                      n138 = call "CheckFile.vi"("Image count filepath"=w476) -> ("Byte Stream File out"=w475:refnum<file>)  [unwired: 10 in]
                      n139 = call "WriteOdorFileheader.vi"("Byte Stream File in"=w475) -> ("Byte Stream File out"=w474:refnum<file>)  [unwired: 10 in]
                    }
                    frame #1 {
                      n140 = Tick Count (ms)() -> (millisecond timer value=w477:u32)
                    }
                  }
                  n141 = local read "Time between trials"() -> (w468:u16)
                  n142 = Array Size(array=w471) -> (size(s)=w470:i32)
                  n143 = Add(x=w468, y=w473) -> (x+y=w469:dbl)
                  n144 = Multiply(x=w469, y=w470) -> (x*y=→"Estimated total time":dbl)
                }
              }
              n145 = local write "Pause elapsed time"(0.0 ("Pause elapsed time")) -> ()
              n146 = local write "In between trials"(FALSE ("In between trials")) -> ()
            }
          }
          n147 = local read "Total trial time"() -> (w350:dbl)
          n148 = Add(x=i8 16, y=w286) -> (x+y=w390:i8)
          n149 = Equal?(x=w286, y="Selected default valve") -> (x = y?=w279:bool)
          n150 = Number To Decimal String(number=w390) -> (decimal integer string=w391:string)  [unwired: 1 in]
          n151 = Select(t=10 ("f"), s=w279, f="Selected default valve") -> (s? t:f=w283:i32)
          n152 = Concatenate Strings("/Dev2/port0/line" ("string"), w391) -> (w307:string)
          n153 = Add(x=i8 16, y=w283) -> (x+y=w304:i32)
          n154 = Number To Decimal String(number=w304) -> (decimal integer string=w303:string)  [unwired: 1 in]
          n155 = Select(t=w282, s=w279, f=w281) -> (s? t:f=w280:u8)
          n156 = Concatenate Strings("/Dev2/port0/line" ("string"), w303) -> (w301:string)
          n157 = case shown="True" "Use Default valve" {
            tunnel: w307 -> [w424 w427]
            tunnel: "/Dev2/port0/line25" ("string") -> [w423 w426]
            tunnel: [w422 w428] -> w305
            tunnel: w301 -> [_ w425]
            frame False {
              n158 = Build Array(w424, w423) -> (w422:string[])
            }
            frame True {
              n159 = Build Array(w427, w425, w426) -> (w428:string[])
            }
          }
          n160 = local read "Valve opening time"() -> (w364:dbl)
          n161 = local read "Valve delay"() -> (w363:dbl)
          n162 = call <vilib>:"DAQmx Flatten Channel String.vi"("names in"=w305) -> ("names out"=w380:string, "error out"=w348:errorcluster)  [unwired: 13 in]
          n163 = call-poly <vilib>:"DAQmx Create Virtual Channel.vi"("edge"=w346, "counter"=tag "Dev2/ctr1") -> ("task out"=w330:refnum<k21>, "error out"=w327:errorcluster)  [unwired: 12 in]
          n164 = Add(x=w363, y=w364) -> (x+y=w394:dbl)
          n165 = call-poly <vilib>:"DAQmx Create Virtual Channel.vi"("frequency"=w315, "duty cycle"=0.5, "counter"=w398) -> ("task out"=w417:refnum<k21>, "error out"=w296:errorcluster)  [unwired: 11 in]
          n166 = call-poly <vilib>:"DAQmx Create Virtual Channel.vi"("lines"=w380, "line grouping"=w414, "error in"=w348) -> ("task out"=w421:refnum<k21>, "error out"=w420:errorcluster)  [unwired: 11 in]
          n167 = Concatenate Strings("/", w398, "InternalOutput" ("string")) -> (w345:string)
          n168 = Subtract(x=w350, y=w394) -> (x-y=w393:dbl)
          n169 = Multiply(x=w315, y=w364) -> (x*y=w396:dbl)
          n170 = Multiply(x=w315, y=w363) -> (x*y=w397:dbl)
          n171 = Subtract(x=w350, y=w379) -> (x-y=w388:dbl)
          n172 = Multiply(x=w315, y=w379) -> (x*y=w384:dbl)
          n173 = To Unsigned Long Integer(number=w397) -> (unsigned 32bit integer=w312:u32)
          n174 = Multiply(x=w315, y=w393) -> (x*y=w395:dbl)
          n175 = To Unsigned Long Integer(number=w396) -> (unsigned 32bit integer=w313:u32)
          n176 = Multiply(x=w315, y=w388) -> (x*y=w386:dbl)
          n177 = To Unsigned Long Integer(number=w384) -> (unsigned 32bit integer=w385:u32)
          n178 = To Unsigned Long Integer(number=w395) -> (unsigned 32bit integer=w314:u32)
          n179 = property class="DAQmx Channel"(reference=w330, error in=w327, "CI.CountEdges.Term"=tag "/Dev2/PFI1") -> (reference out=w329:refnum<k21>, error out=w328:errorcluster)
          n180 = To Unsigned Long Integer(number=w386) -> (unsigned 32bit integer=w387:u32)
          n181 = property class="DAQmx Channel"(reference=w417, error in=w296, "CO.Pulse.Term"=tag "/Dev2/PFI12") -> (reference out=w297:refnum<k21>, error out=w295:errorcluster)
          n182 = call-poly <vilib>:"Digital Pattern Generator.vi"("value"=w382, "sample rate"=w315, "number of signals"=w381, "number of samples"=w385) -> ("digital waveform"=w367:digitalwaveform)  [unwired: 6 in, 1 out]
          n183 = call-poly <vilib>:"Digital Pattern Generator.vi"("value"=w318, "sample rate"=w315, "number of signals"=w316, "number of samples"=w313) -> ("digital waveform"=w323:digitalwaveform)  [unwired: 6 in, 1 out]
          n184 = call-poly <vilib>:"Digital Pattern Generator.vi"("value"=w317, "sample rate"=w315, "number of signals"=w316, "number of samples"=w312) -> ("digital waveform"=w324:digitalwaveform)  [unwired: 6 in, 1 out]
          n185 = call-poly <vilib>:"Digital Pattern Generator.vi"("value"=w406, "sample rate"=w315, "number of signals"=w405, "number of samples"=w313) -> ("digital waveform"=w372:digitalwaveform)  [unwired: 6 in, 1 out]
          n186 = call-poly <vilib>:"Digital Pattern Generator.vi"("value"=w280, "sample rate"=w315, "number of signals"=w405, "number of samples"=w312) -> ("digital waveform"=w371:digitalwaveform)  [unwired: 6 in, 1 out]
          n187 = Compound Arithmetic op=ADD(w364, w363, 10.0 ("Wert")) -> (w365:dbl)
          n188 = property on="Digitaler output" class="DigitalGraph (strict)"("XScale.Maximum"=w365) -> ()  [unwired: 2 in, 2 out]
          n189 = call-poly <vilib>:"Digital Pattern Generator.vi"("value"=w383, "sample rate"=w315, "number of signals"=w381, "number of samples"=w387) -> ("digital waveform"=w368:digitalwaveform)  [unwired: 6 in, 1 out]
          n190 = property on="Digital Waveform Graph" class="DigitalGraph (strict)"("XScale.Maximum"=w365) -> ()  [unwired: 2 in, 2 out]
          n191 = call-poly <vilib>:"Digital Pattern Generator.vi"("value"=w319, "sample rate"=w315, "number of signals"=w316, "number of samples"=w314) -> ("digital waveform"=w326:digitalwaveform)  [unwired: 6 in, 1 out]
          n192 = call-poly <vilib>:"Append Digital Samples.vi"("digital waveform B"=w323, "digital waveform A"=w324) -> ("digital waveform out"=w325:digitalwaveform)  [unwired: 8 in, 1 out]
          n193 = call-poly <vilib>:"Digital Pattern Generator.vi"("value"=w280, "sample rate"=w315, "number of signals"=w405, "number of samples"=w314) -> ("digital waveform"=w369:digitalwaveform)  [unwired: 6 in, 1 out]
          n194 = call-poly <vilib>:"Append Digital Samples.vi"("digital waveform B"=w372, "digital waveform A"=w371) -> ("digital waveform out"=w370:digitalwaveform)  [unwired: 8 in, 1 out]
          n195 = disable-structure shown="Enabled" {
            disable-tunnel: w329 -> [w443 w445]
            disable-tunnel: w315 -> [w442 _]
            disable-tunnel: w345 -> [w441 _]
            disable-tunnel: w328 -> [w440 w444]
            disable-tunnel: [w439 w445] -> w344
            disable-tunnel: [w438 w444] -> w291
            disable-tunnel: w293 -> [w437 _]
            frame Enabled {
              n196 = call-poly <vilib>:"DAQmx Timing.vi"("task/channels in"=w443, "sample mode"=w437, "rate"=w442, "source"=w441, "error in"=w440) -> ("task out"=w439:refnum<k21>, "error out"=w438:errorcluster)  [unwired: 9 in]
            }
            frame Disabled {
            }
          }
          n197 = Multiply(x=w350, y=w315) -> (x*y=w288:dbl)
          n198 = call-poly <vilib>:"Append Digital Samples.vi"("digital waveform B"=w368, "digital waveform A"=w367) -> ("digital waveform out"=w378:digitalwaveform)  [unwired: 8 in, 1 out]
          n199 = call-poly <vilib>:"DAQmx Timing.vi"("task/channels in"=w421, "sample mode"=w289, "samples per channel"=w288, "rate"=w315, "source"=w345, "error in"=w420) -> ("task out"=w411:refnum<k21>, "error out"=w410:errorcluster)  [unwired: 8 in]
          n200 = call-poly <vilib>:"Append Digital Samples.vi"("digital waveform B"=w326, "digital waveform A"=w325) -> ("digital waveform out"=w320:digitalwaveform)  [unwired: 8 in, 1 out]
          n201 = call-poly <vilib>:"Append Digital Samples.vi"("digital waveform B"=w369, "digital waveform A"=w370) -> ("digital waveform out"=w375:digitalwaveform)  [unwired: 8 in, 1 out]
          n202 = call-poly <vilib>:"DAQmx Timing.vi"("task/channels in"=w297, "sample mode"=w293, "error in"=w295) -> ("task out"=w415:refnum<k21>, "error out"=w416:errorcluster)  [unwired: 11 in]
          n203 = Set Waveform Attribute(5:"Scanimage trigger", 6:"NI_LineNames" ("name"), 7:w378) -> (3:w309:digitalwaveform)  [unwired: 1 in, 2 out]
          n204 = Set Waveform Attribute(5:"Default Valve signal", 6:"NI_LineNames" ("name"), 7:w320) -> (3:w308:digitalwaveform)  [unwired: 1 in, 2 out]
          n205 = Set Waveform Attribute(5:"Valve signal", 6:"NI_LineNames" ("name"), 7:w375) -> (3:w310:digitalwaveform)  [unwired: 1 in, 2 out]
          n206 = case shown="False" "Use Default valve" {
            tunnel: w310 -> [w431 w436]
            tunnel: w309 -> [w430 w434]
            tunnel: [w429 w435] -> w311
            tunnel: w308 -> [_ w433]
            frame False {
              n207 = call-poly <vilib>:"Append Digital Signals.vi"("digital waveform (low bits)"=w430, "digital waveform (high bits)"=w431) -> ("digital waveform out"=w429:digitalwaveform)  [unwired: 8 in, 1 out]
            }
            frame True {
              n208 = call-poly <vilib>:"Append Digital Signals.vi"("digital waveform (low bits)"=w434, "digital waveform (high bits)"=w433) -> ("digital waveform out"=w432:digitalwaveform)  [unwired: 8 in, 1 out]
              n209 = call-poly <vilib>:"Append Digital Signals.vi"("digital waveform (low bits)"=w432, "digital waveform (high bits)"=w436) -> ("digital waveform out"=w435:digitalwaveform)  [unwired: 8 in, 1 out]
            }
          }
          n210 = call-poly <vilib>:"DAQmx Write.vi"("task/channels in"=w411, "auto start"=FALSE, "data"=w311, "error in"=w410) -> ("task out"=w409:refnum<k21>, "error out"=w408:errorcluster)  [unwired: 9 in, 1 out]
          n211 = call <vilib>:"DAQmx Start Task.vi"("task/channels in"=w344, "error in"=w291) -> ("task out"=w292:refnum<k21>, "error out"=w290:errorcluster)  [unwired: 12 in]
          n212 = call <vilib>:"DAQmx Start Task.vi"("task/channels in"=w409, "error in"=w408) -> ("task out"=w413:refnum<k21>, "error out"=w412:errorcluster)  [unwired: 12 in]
          n213 = flat-sequence {
            tunnel: [w584] -> w419
            tunnel: [w583] -> w418
            tunnel: w416 -> [w582]
            tunnel: w415 -> [w585]
            tunnel: [w594] -> w404
            tunnel: w413 -> [w594]
            tunnel: [w593] -> w403
            tunnel: w412 -> [w593]
            tunnel: [w592] -> w356
            tunnel: w292 -> [w591]
            tunnel: w290 -> [w590]
            tunnel: [w591] -> w343
            tunnel: [w590] -> w342
            tunnel: bool[] [FALSE, FALSE, FALSE] ("data") -> [w589]
            tunnel: [w589] -> w340
            tunnel: [w588] -> w338
            tunnel: w339 -> [w588]
            tunnel: [w587] -> w336
            tunnel: w305 -> [w587]
            tunnel: [w586] -> w335
            tunnel: w286 -> [w586]
            frame #0 {
              n214 = Tick Count (ms)() -> (millisecond timer value=w592:u32)
              n215 = call <vilib>:"DAQmx Start Task.vi"("task/channels in"=w585, "error in"=w582) -> ("task out"=w584:refnum<k21>, "error out"=w583:errorcluster)  [unwired: 12 in]
            }
          }
          n216 = call-poly <vilib>:"Digital to Boolean Array.vi"("digital waveform"=w311) -> ()  [unwired: 9 in, 2 out]
          n217 = disable-structure shown="Aktiviert" {
            disable-tunnel: w419 -> [w526 _]
            disable-tunnel: w418 -> [w525 _]
            disable-tunnel: [w524 _] -> w360
            disable-tunnel: [w523 _] -> w361
            disable-tunnel: w404 -> [w522 _]
            disable-tunnel: w403 -> [w521 _]
            disable-tunnel: [w520 _] -> w402
            disable-tunnel: [w519 _] -> w355
            disable-tunnel: w356 -> [w518 _]
            disable-tunnel: w349 -> [w517 _]
            disable-tunnel: w343 -> [w507 _]
            disable-tunnel: w342 -> [w516 _]
            disable-tunnel: w340 -> [w515 _]
            disable-tunnel: w338 -> [w514 _]
            disable-tunnel: [w513 _] -> w337
            disable-tunnel: w336 -> [w512 _]
            disable-tunnel: w335 -> [w511 _]
            disable-tunnel: [w510 _] -> w333
            disable-tunnel: [w509 _] -> w331
            disable-tunnel: [w508 _] -> w298
            frame Enabled {
              n218 = while {
                shift-right: [w562] -> w523
                shift-left: w526 -> [w564]
                shift-right: [w561] -> w524
                shift-left: w525 -> [w563]
                tunnel: w522 -> [w560]
                tunnel: w521 -> [w545]
                tunnel: [w530] -> w520
                tunnel: [w528] -> w519
                tunnel: w518 -> [w555]
                tunnel: w517 -> [w552]
                tunnel: w507 -> [w544]
                tunnel: w516 -> [w542]
                tunnel: [w543] -> w508
                tunnel: [w541] -> w513
                shift-right: [w537] -> _
                shift-left: w515 -> [w540]
                shift-right: [w534] -> w510
                shift-left: w514 -> [w535]
                tunnel: w512 -> [w533]
                tunnel: w511 -> [w532]
                tunnel: [w531] -> w509
                stop <- w556 stop-if-true
                n219 = call-poly <vilib>:"DAQmx Read.vi"("task/channels in"=w544, "error in"=w542) -> ("task out"=w543:refnum<k21>, "data"=w536:u32, "error out"=w541:errorcluster)  [unwired: 11 in]
                "Framecount" <- w536
                n220 = call-poly <vilib>:"DAQmx Read.vi"("task/channels in"=w560, "error in"=w545) -> ("task out"=w546:refnum<k21>, "data"=w537:bool[], "error out"=w529:errorcluster)  [unwired: 11 in]
                n221 = Not Equal?(x=w537, y=w540) -> (x != y?=w539:bool[])
                n222 = Or Array Elements(Boolean array=w539) -> (logical OR=w538:bool)
                n223 = Tick Count (ms)() -> (millisecond timer value=w553:u32)
                n224 = case shown="True" w538 {
                  tunnel: w537 -> [_ w578]
                  tunnel: w536 -> [_ w576]
                  tunnel: w535 -> [w567 w580]
                  tunnel: [w567 w579] -> w534
                  tunnel: w533 -> [_ w570]
                  tunnel: w532 -> [_ w573]
                  tunnel: [errorcluster {"status"=FALSE, "code"=0, "source"=""} ("error out") w569] -> w531
                  frame False {
                  }
                  frame True {
                    w571 = "\t"
                    n225 = Boolean To (0,1)(Boolean=w578) -> (0, 1=w577:i16[])
                    n226 = Number To Decimal String(number=w577) -> (decimal integer string=w574:string[])  [unwired: 1 in]
                    n227 = Number To Decimal String(number=w576) -> (decimal integer string=w575:string)  [unwired: 1 in]
                    n228 = Number To Decimal String(number=w573) -> (decimal integer string=w572:string)  [unwired: 1 in]
                    n229 = Concatenate Strings(w575, w571, w574, w571, w572, w571, w570, "\r\n") -> (w581:string)
                    n230 = Write to Text File(file (use dialog)=w580, text=w581) -> (refnum out=w579:refnum<file>, error out=w569:errorcluster)  [unwired: 2 in, 1 out]
                  }
                }
                n231 = Wait (ms)(milliseconds to wait=u32 1 ("Zu wartende ms")) -> ()  [unwired: 1 out]
                n232 = call <vilib>:"DAQmx Is Task Done.vi"("task/channels in"=w546, "error in"=w529) -> ("task out"=w530:refnum<k21>, "task done?"=w527:bool, "error out"=w528:errorcluster)  [unwired: 11 in]
                n233 = Subtract(x=w553, y=w555) -> (x-y=w548:u32)
                n234 = local read "Stop Boolesch"() -> (w557:bool)
                n235 = call <vilib>:"DAQmx Is Task Done.vi"("task/channels in"=w564, "error in"=w563) -> ("task out"=w562:refnum<k21>, "error out"=w561:errorcluster)  [unwired: 11 in, 1 out]
                n236 = Subtract(x=w553, y=w552) -> (x-y=w550:u32)
                n237 = Divide(x=w548, y=u32 1000 ("x")) -> (x/y=→"Trial elapsed time":dbl)
                n238 = Unbundle By Name(w528) -> ("status"=w558:bool)
                n239 = Divide(x=w550, y=u32 1000 ("x")) -> (x/y=→"Total elapsed time":dbl)
                n240 = Or(x=w558, y=w557) -> (x .or. y?=w565:bool)
                n241 = Or(x=w527, y=w565) -> (x .or. y?=w556:bool)
              }
            }
            frame Disabled {
            }
          }
          n242 = local write "Digital Waveform Graph"(w311) -> ()
          n243 = local write "Digitaler output"(w311) -> ()
          n244 = disable-structure shown="Enabled" {
            disable-tunnel: w402 -> [w449 w451]
            disable-tunnel: [w448 w451] -> w359
            disable-tunnel: w355 -> [w447 w450]
            disable-tunnel: [w446 w450] -> w354
            frame Enabled {
              n245 = call <vilib>:"DAQmx Wait Until Done.vi"("task/channels in"=w449, "error in"=w447) -> ("task out"=w448:refnum<k21>, "error out"=w446:errorcluster)  [unwired: 12 in]
            }
            frame Disabled {
            }
          }
          n246 = flat-sequence {
            tunnel: w361 -> [w491]
            tunnel: w360 -> [w480]
            tunnel: w359 -> [w490]
            tunnel: w354 -> [w482]
            tunnel: w337 -> [w485]
            tunnel: w298 -> [w488]
            tunnel: w349 -> [w494]
            frame #0 {
              n247 = call <vilib>:"DAQmx Stop Task.vi"("task/channels in"=w488, "error in"=w485) -> ("task out"=w487:refnum<k21>, "error out"=w486:errorcluster)  [unwired: 12 in]
              n248 = call <vilib>:"DAQmx Stop Task.vi"("task/channels in"=w490, "error in"=w482) -> ("task out"=w483:refnum<k21>, "error out"=w481:errorcluster)  [unwired: 12 in]
              n249 = call <vilib>:"DAQmx Stop Task.vi"("task/channels in"=w491, "error in"=w480) -> ("task out"=w484:refnum<k21>, "error out"=w479:errorcluster)  [unwired: 12 in]
              n250 = call <vilib>:"DAQmx Clear Task.vi"("task in"=w487, "error in"=w486) -> ("error out"=w489:errorcluster)  [unwired: 13 in]
              n251 = call <vilib>:"DAQmx Clear Task.vi"("task in"=w484, "error in"=w479) -> ("error out"=w492:errorcluster)  [unwired: 13 in]
              n252 = call <vilib>:"DAQmx Clear Task.vi"("task in"=w483, "error in"=w481) -> ("error out"=w493:errorcluster)  [unwired: 13 in]
              n253 = Merge Errors(w492, w493, w489) -> ()  [unwired: 1 out]
            }
            frame #1 {
              n254 = Tick Count (ms)() -> (millisecond timer value=w495:u32)
              n255 = for {
                N: "Time between trials" -> [_]
                tunnel: w495 -> [w505]
                tunnel: w494 -> [w500]
                stop <- w498 stop-if-true
                w502 = u32 1000 ("Zu wartende ms")
                n256 = Tick Count (ms)() -> (millisecond timer value=w499:u32)
                n257 = Subtract(x=w499, y=w505) -> (x-y=w506:u32)
                n258 = Subtract(x=w499, y=w500) -> (x-y=w503:u32)
                n259 = local read "Stop Boolesch"() -> (w498:bool)
                n260 = Divide(x=w506, y=w502) -> (x/y=→"Pause elapsed time":dbl)
                n261 = Divide(x=w503, y=w502) -> (x/y=w501:dbl)
                n262 = local write "Total elapsed time"(w501) -> ()
                n263 = Wait (ms)(milliseconds to wait=w502) -> ()  [unwired: 1 out]
              }
              "In between trials" <- TRUE ("In between trials")
            }
          }
          n264 = local read "Stop Boolesch"() -> (w362:bool)
          "Current Valve" <- w353
          "Current list index" <- w358
        }
        n265 = local write "Experiment running"(TRUE ("Experiment running")) -> ()
        n266 = Close File(refnum=w271, error in=w270) -> ()  [unwired: 2 out]
        "State" <- w276
      }
      frame "Stop" {
        n267 = local write "State"(w595) -> ()
        n268 = flat-sequence {
          frame #0 {
            # "Stop-all to zero"
            # "all lines also trigger line"
            n269 = call-poly <vilib>:"DAQmx Write.vi"("task/channels in"="/Dev2/port0/line17:25" ("string"), "data"=bool[] [FALSE, FALSE, FALSE, FALSE, FALSE, FALSE, FALSE, FALSE, FALSE]) -> ("task out"=w603:refnum<k21>, "error out"=w598:errorcluster)  [unwired: 11 in, 1 out]
            n270 = call <vilib>:"DAQmx Start Task.vi"("task/channels in"=w603, "error in"=w598) -> ("task out"=w602:refnum<k21>, "error out"=w600:errorcluster)  [unwired: 12 in]
            n271 = call <vilib>:"DAQmx Wait Until Done.vi"("task/channels in"=w602, "error in"=w600) -> ("task out"=w601:refnum<k21>, "error out"=w599:errorcluster)  [unwired: 12 in]
            n272 = call <vilib>:"DAQmx Clear Task.vi"("task in"=w601, "error in"=w599) -> ()  [unwired: 13 in, 1 out]
          }
          frame #1 {
            w606 = T2."Enabled" ("Deaktiviert")
            n273 = property on="Select experiment" class="TabCtl (strict)"() -> ("Pages"=w609:refnum<vi>[])  [unwired: 2 in, 2 out]
            n274 = property on="Valve order list" class="Arr (strict)"("DisabledEnum"=T2."Enabled" ("Deaktiviert")) -> ()  [unwired: 2 in, 2 out]
            n275 = for {
              tunnel: w609 -> [w610] mode=indexing
              n276 = property class="Page"(reference=w610, "PageEnb"=T3."Page Enabled" ("Aktiv-Status der Seite")) -> ()  [unwired: 1 in, 2 out]
            }
            n277 = property on="Start trial series" class="Bool"("DisabledEnum"=w606) -> ()  [unwired: 2 in, 2 out]
            n278 = property on="Start single trial" class="Bool"("DisabledEnum"=w606) -> ()  [unwired: 2 in, 2 out]
            n279 = property on="Image count filepath" class="Path"("DisabledEnum"=w606) -> ()  [unwired: 2 in, 2 out]
            "Experiment running" <- FALSE ("Experiment running")
          }
        }
        n280 = local read "Stop Boolesch"() -> (w597:bool)
      }
    }
  }
  n281 = while {
    tunnel: w4 -> [w613]
    stop <- w612 stop-if-true
    n282 = event shown="[3] \"Load exp. ini\": Value Change" {
      selector: _ -> [_ _ _ _ _]
      dyn-events: _ -> [_ _ _ _ _]
      timeout: _ -> [_ _ _ _ _]
      tunnel: w613 -> [_ w614 w623 _ w678]
      event Timeout {
        n283 = event-data() -> ()  [unwired: 1 in, 3 out]
      }
      event "Start single trial": Value Change {
        n284 = event-data() -> ()  [unwired: 1 in, 6 out]
        n285 = case shown="True" "Start single trial" {
          tunnel: w614 -> [_ w622]
          frame False {
          }
          frame True {
            n286 = property on="Start single trial" class="Bool"("DisabledEnum"=T2."Disabled and Grayed Out" ("Deaktiviert")) -> ()  [unwired: 2 in, 2 out]
            n287 = Enqueue Element(queue=w622, element=StatesEnum."Start Trial" ("Enum")) -> ()  [unwired: 2 in, 3 out]
            n288 = property on="Select experiment" class="TabCtl (strict)"() -> ("Pages"=w618:refnum<vi>[])  [unwired: 2 in, 2 out]
            n289 = Index Array(array=w618, index=1 ("Index")) -> (element=w619:refnum<vi>)
            n290 = property class="Page"(reference=w619, "PageEnb"=T3."Page Disabled & Grayed" ("Aktiv-Status der Seite")) -> ()  [unwired: 1 in, 2 out]
          }
        }
      }
      event "Stopp": Value Change {
        n291 = event-data() -> ()  [unwired: 1 in, 6 out]
        n292 = case shown="True" "Stopp" {
          tunnel: w623 -> [_ w627]
          frame False {
          }
          frame True {
            n293 = Enqueue Element(queue=w627, element=StatesEnum."Stop" ("Enum")) -> ()  [unwired: 2 in, 3 out]
            "Stop Boolesch" <- TRUE ("Stop Boolesch")
          }
        }
      }
      event "Load exp. ini": Value Change {
        n294 = event-data() -> ()  [unwired: 1 in, 6 out]
        n295 = case shown="True" "Load exp. ini" {
          frame False {
          }
          frame True {
            n296 = call "File Dialog"("prompt"="Please select an experiment ini file", "pattern (all files)"="*.ini") -> ("selected path"=w629:path, "cancelled"=w630:bool)  [unwired: 10 in, 2 out]
            n297 = case shown="False" w630 {
              tunnel: w629 -> [w671 _]
              frame False {
                w643 = "Odor System" ("section")
                n298 = call <vilib>:"Open Config Data.vi"("configuration file path"=w671) -> ("error out"=w669:errorcluster, "refnum"=w670:T4)  [unwired: 8 in, 1 out]
                n299 = call-poly <vilib>:"Read Key.vi"("section"=w643, "error in (no error)"=w669, "key"="Value delay", "refnum"=w670) -> ("error out"=w665:errorcluster, "value"=w667:dbl, "refnum out"=w666:T4)  [unwired: 4 in, 1 out]
                n300 = local write "Valve delay"(w667) -> ()
                n301 = call-poly <vilib>:"Read Key.vi"("section"=w643, "error in (no error)"=w665, "key"="Valve opening time", "refnum"=w666) -> ("error out"=w661:errorcluster, "value"=w663:dbl, "refnum out"=w662:T4)  [unwired: 4 in, 1 out]
                n302 = local write "Valve opening time"(w663) -> ()
                n303 = call-poly <vilib>:"Read Key.vi"("section"=w643, "error in (no error)"=w661, "key"="Total trial time", "refnum"=w662) -> ("error out"=w658:errorcluster, "value"=w659:dbl, "refnum out"=w657:T4)  [unwired: 4 in, 1 out]
                n304 = local write "Total trial time"(w659) -> ()
                n305 = call-poly <vilib>:"Read Key.vi"("section"=w643, "error in (no error)"=w658, "key"="Time between trials", "refnum"=w657) -> ("error out"=w654:errorcluster, "value"=w653:i32, "refnum out"=w655:T4)  [unwired: 4 in, 1 out]
                n306 = local write "Time between trials"(w653) -> ()
                n307 = call-poly <vilib>:"Read Key.vi"("section"=w643, "error in (no error)"=w654, "key"="Use Default valve", "refnum"=w655) -> ("error out"=w649:errorcluster, "value"=w651:bool, "refnum out"=w650:T4)  [unwired: 4 in, 1 out]
                n308 = local write "Use Default valve"(w651) -> ()
                n309 = call-poly <vilib>:"Read Key.vi"("section"=w643, "error in (no error)"=w649, "key"="Selected default valve ", "refnum"=w650) -> ("error out"=w645:errorcluster, "value"=w647:i32, "refnum out"=w646:T4)  [unwired: 4 in, 1 out]
                n310 = local write "Selected default valve"(w647) -> ()
                n311 = call-poly <vilib>:"Read Key.vi"("section"=w643, "error in (no error)"=w645, "key"="Valve order list", "refnum"=w646) -> ("error out"=w638:errorcluster, "value"=w642:string, "refnum out"=w639:T4)  [unwired: 4 in, 1 out]
                n312 = Spreadsheet String To Array(delimiter (Tab)=";", format string="%d", spreadsheet string=w642, array type (2D Dbl)=i8[] [] ("Valve order list")) -> (array=w640:i8[])
                n313 = local write "Valve order list"(w640) -> ()
                n314 = call <vilib>:"Close Config Data.vi"("error in (no error)"=w638, "refnum"=w639) -> ("error out"=w636:errorcluster, "file path"=w635:path)  [unwired: 8 in]
                n315 = Unbundle By Name(w636) -> ("status"=w637:bool)
                n316 = case shown="True" w637 {
                  tunnel: w636 -> [_ w676]
                  tunnel: w635 -> [w673 _]
                  frame False {
                    n317 = Strip Path(path=w673) -> (name=→"Loaded experiment":string)  [unwired: 1 out]
                  }
                  frame True {
                    w675 = T5 3 items=["no dialog", "OK message", "continue or stop message", "OK message + warnings", "continue/stop + warnings"] ("type of dialog (OK msg:1)")
                    n318 = call <vilib>:"Simple Error Handler.vi"("error source (\" \")"="Error loading experiment ini file" ("error source (\" \")"), "type of dialog (OK msg:1)"=w675, "error in (no error)"=w676) -> ()  [unwired: 2 in, 5 out]
                  }
                }
              }
              frame True {
              }
            }
          }
        }
      }
      event "Start trial series": Value Change {
        n319 = event-data() -> ()  [unwired: 1 in, 6 out]
        n320 = case shown="True" "Start trial series" {
          tunnel: w678 -> [_ w685]
          frame False {
          }
          frame True {
            n321 = property on="Start trial series" class="Bool"("DisabledEnum"=T2."Disabled and Grayed Out" ("Deaktiviert")) -> ()  [unwired: 2 in, 2 out]
            n322 = Enqueue Element(queue=w685, element=StatesEnum."Start trial series" ("Enum")) -> ()  [unwired: 2 in, 3 out]
            n323 = property on="Select experiment" class="TabCtl (strict)"() -> ("Pages"=w681:refnum<vi>[])  [unwired: 2 in, 2 out]
            n324 = Index Array(array=w681, index=0 ("Index")) -> (element=w682:refnum<vi>)
            n325 = property class="Page"(reference=w682, "PageEnb"=T3."Page Disabled & Grayed" ("Aktiv-Status der Seite")) -> ()  [unwired: 1 in, 2 out]
          }
        }
      }
    }
    n326 = local read "Stop Boolesch"() -> (w612:bool)
  }
  n327 = Release Queue(queue=w3) -> ()  [unwired: 2 in, 3 out]
